vi "Define Default Prefix.vi"(8 "error in":errorcluster, 11 "AI channel in":refnum<class "AI Channel.lvclass">) -> (0 "error out":errorcluster, 3 "AI channel out":refnum<class "AI Channel.lvclass">)   [LabVIEW 2020, in "Scan Engine Scripting.lvlib" / "AI Channel.lvclass"]
uses:
  AI Channel.lvclass
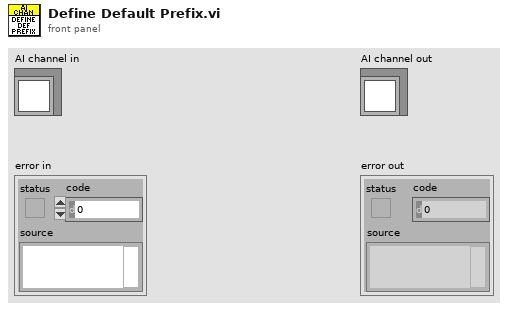
[diagram p1: front panel]
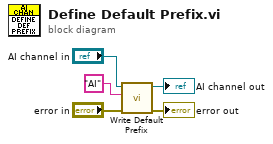
[diagram p0: block diagram]
diagram:
  n1 = call-dynamic "Write Default Prefix.vi"("error in"="error in", "default prefix"="AI", "channel in"="AI channel in") -> ("error out"=→"error out":errorcluster, "channel out"=→"AI channel out":refnum<class "AI Channel.lvclass">)  [unwired: 7 in]
